vi "HFRR ADV v028 new software.vi"() -> ()   [LabVIEW 2025] (continued)
                      }
                      frame #27 {
                        n2418 = local read "Set Temp"() -> (w3472:dbl)
                        n2419 = Number To Fractional String(number=w3472, precision (6)=i16 2) -> (F-format string=w3473:string)  [unwired: 2 in]
                        n2420 = Concatenate Strings("Set Temperature [deg C] :" ("Content"), w3473) -> (w3475:string)
                        n2421 = local read "EVENT LOG"() -> (w3477:string)
                        n2422 = call "Event Log.vi"("Content"=w3475, "EVENT LOG"=w3477) -> ("EVENT LOG"=w3476:string)  [unwired: 8 in, 1 out]
                        n2423 = local write "EVENT LOG"(w3476) -> ()
                      }
                      frame #28 {
                        n2424 = Wait (ms)(milliseconds to wait=u32 50) -> ()  [unwired: 1 out]
                      }
                      frame #29 {
                        n2425 = local read "Set Rh"() -> (w3480:dbl)
                        n2426 = Number To Fractional String(number=w3480, precision (6)=i16 2) -> (F-format string=w3481:string)  [unwired: 2 in]
                        n2427 = Concatenate Strings("Set Humidity [%RH] :" ("Content"), w3481) -> (w3483:string)
                        n2428 = local read "EVENT LOG"() -> (w3485:string)
                        n2429 = call "Event Log.vi"("Content"=w3483, "EVENT LOG"=w3485) -> ("EVENT LOG"=w3484:string)  [unwired: 8 in, 1 out]
                        n2430 = local write "EVENT LOG"(w3484) -> ()
                      }
                      frame #30 {
                        n2431 = Wait (ms)(milliseconds to wait=u32 50) -> ()  [unwired: 1 out]
                      }
                      frame #31 {
                        n2432 = local read "test time"() -> (w3488:dbl)
                        n2433 = Number To Fractional String(number=w3488, precision (6)=i16 1) -> (F-format string=w3489:string)  [unwired: 2 in]
                        n2434 = Concatenate Strings("Test Duration [mins] :" ("Content"), w3489) -> (w3491:string)
                        n2435 = local read "EVENT LOG"() -> (w3493:string)
                        n2436 = call "Event Log.vi"("Content"=w3491, "EVENT LOG"=w3493) -> ("EVENT LOG"=w3492:string)  [unwired: 8 in, 1 out]
                        n2437 = local write "EVENT LOG"(w3492) -> ()
                      }
                      frame #32 {
                        w3494 = dbl[] [] ("History Data")
                        w3495 = cluster{"y":dbl, dbl, "y":dbl}[] [] ("History Data")
                        w3496 = FALSE ("Visible")
                        n2438 = property on="Stroke ( mm )" class="WFChart (strict)"("History Data"=w3495) -> ()  [unwired: 2 in, 2 out]
                        n2439 = property on="Humidity ( %RH )" class="WFChart (strict)"("History Data"=w3494) -> ()  [unwired: 2 in, 2 out]
                        n2440 = property on="Temperature ( Deg C )" class="WFChart (strict)"("History Data"=w3494) -> ()  [unwired: 2 in, 2 out]
                        n2441 = property on="Electrical Contact Resistance ( % )" class="WFChart (strict)"("History Data"=w3494) -> ()  [unwired: 2 in, 2 out]
                        n2442 = property on="Coefficient of Friction" class="WFChart (strict)"("History Data"=w3494) -> ()  [unwired: 2 in, 2 out]
                        n2443 = property on="Frictional Force ( N )" class="WFChart (strict)"("History Data"=w3494) -> ()  [unwired: 2 in, 2 out]
                        n2444 = property on="Coefficient of Friction" class="WFChart (strict)"("History Data"=w3494) -> ()  [unwired: 2 in, 2 out]
                        n2445 = property on="Frictional Force ( N )" class="WFChart (strict)"("History Data"=w3494) -> ()  [unwired: 2 in, 2 out]
                        n2446 = property on="Electrical Contact Resistance ( % )" class="WFChart (strict)"("History Data"=w3494) -> ()  [unwired: 2 in, 2 out]
                        n2447 = property on="Humidity ( %RH )" class="WFChart (strict)"("History Data"=w3494) -> ()  [unwired: 2 in, 2 out]
                        n2448 = property on="Stroke ( mm )" class="WFChart (strict)"("History Data"=w3495) -> ()  [unwired: 2 in, 2 out]
                        n2449 = property on="Temperature ( Deg C )" class="WFChart (strict)"("History Data"=w3494) -> ()  [unwired: 2 in, 2 out]
                        n2450 = property on="Service Password Log" class="Str"("Visible"=w3496) -> ()  [unwired: 2 in, 2 out]
                        n2451 = property on="Password 3" class="Clust (strict)"("Visible"=w3496) -> ()  [unwired: 2 in, 2 out]
                      }
                    }
                    "TEST FILE NAM,E SAVED" <- TRUE ("TEST FILE NAM,E SAVED")
                  }
                }
              }
            }
          }
        }
        n2452 = local write "Test \nStatus"(w2886) -> ()
        n2453 = local write "Save"(w2886) -> ()
        n2454 = local read "Main Tab"() -> (w2880:T2)
        n2455 = case shown="True" w2883 {
          frame False {
            n2456 = local read "Rt 3"() -> (w2955:bool)
            n2457 = case shown="True" w2955 {
              frame False {
              }
              frame True {
                n2458 = local write "Rt 3"(FALSE ("Rt 3")) -> ()
              }
            }
            "Rt" <- TRUE ("Rt")
            "Rt 2" <- FALSE ("Rt")
          }
          frame True {
            n2459 = local read "Rt"() -> (w2961:bool)
            n2460 = local write "Rt 2"(TRUE ("Rt 2")) -> ()
            n2461 = case shown="True" w2961 {
              frame False {
              }
              frame True {
                n2462 = local write "Rt"(FALSE ("Rt")) -> ()
              }
            }
            "Rt 3" <- TRUE ("Rt 3")
          }
        }
        n2463 = case shown="\"Acquire\"" w2880 {
          tunnel: w2882 -> [_ w2989]
          frame Default {
            w2988 = 0.0 ("output")
            n2464 = local write "PID-out"(w2988) -> ()
            n2465 = local write "Frequency ( Hz )"(w2988) -> ()
          }
          frame "Acquire" {
            n2466 = stacked-sequence {
              frame #0 {
                n2467 = local read "Auto Start Test"() -> (w2991:bool)
                n2468 = case shown="True" w2991 {
                  tunnel: "RUN" -> [w3012 w3015]
                  tunnel: [w3012 w3014] -> w2992
                  frame False {
                  }
                  frame True {
                    n2469 = local read "Auto Start Temp"() -> (w3013:bool)
                    n2470 = Or(x=w3015, y=w3013) -> (x .or. y?=w3014:bool)
                  }
                }
                n2471 = local read "clk"() -> (w3011:dbl)
                n2472 = local read "Save"() -> (w3007:bool)
                n2473 = Equal?(x=w3011, y=0.0) -> (x = y?=w3008:bool)
                n2474 = And(x=w3008, y=w3007) -> (x .and. y?=w3009:bool)
                n2475 = Not(x="Engage") -> (.not. x?=w2998:bool)
                n2476 = case shown="False" w2992 {
                  tunnel: [0.0 w3038] -> w2994
                  frame False {
                    (unwired) TRUE ("Visible")
                    n2477 = local read "Auto Start Test"() -> (w3019:bool)
                    n2478 = local write "Start Time"(TRUE ("Start Time")) -> ()
                    n2479 = property on="Stroke 2" class="DigNum (strict)"("Visible"=FALSE) -> ()  [unwired: 2 in, 2 out]
                    n2480 = case shown="False" w3019 {
                      frame False {
                        n2481 = property on="Heater Button" class="Bool (strict)"("DisabledEnum"=T19."Enabled" ("Disabled")) -> ()  [unwired: 2 in, 2 out]
                        n2482 = property on="Humidity" class="Bool (strict)"("DisabledEnum"=T19."Enabled" ("Disabled")) -> ()  [unwired: 2 in, 2 out]
                      }
                      frame True {
                      }
                    }
                    n2483 = case shown="False" "TestCompFlg" {
                      frame False {
                        n2484 = local read "StartFlg"() -> (w3027:bool)
                        n2485 = case shown="True" w3027 {
                          frame False {
                          }
                          frame True {
                            n2486 = stacked-sequence {
                              frame #0 {
                                n2487 = local read "EVENT LOG"() -> (w3031:string)
                                n2488 = call "Event Log.vi"("Content"="Test was interrupted", "EVENT LOG"=w3031) -> ("EVENT LOG"=w3032:string)  [unwired: 8 in, 1 out]
                                n2489 = local write "EVENT LOG"(w3032) -> ()
                                n2490 = property on="RUN" class="Bool (strict)"("Visible"=TRUE) -> ()  [unwired: 2 in, 2 out]
                                n2491 = property on="Auto Start Test" class="Bool (strict)"("Visible"=TRUE) -> ()  [unwired: 2 in, 2 out]
                              }
                              frame #1 {
                                w3034 = FALSE ("StartFlg")
                                n2492 = property on="Heater Button" class="Bool (strict)"("Val(Sgnl)"=FALSE ("Value (Signaling)")) -> ()  [unwired: 2 in, 2 out]
                                n2493 = local write "Heater Button"(w3034) -> ()
                                n2494 = local write "StartFlg"(w3034) -> ()
                                n2495 = local write "Humidity"(w3034) -> ()
                              }
                              frame #2 {
                                n2496 = local write "Due Write"("VC;0" ("Command")) -> ()
                              }
                              frame #3 {
                                n2497 = Wait (ms)(milliseconds to wait=u32 1500) -> ()  [unwired: 1 out]
                              }
                              frame #4 {
                                n2498 = local write "Due Write"("HE;0" ("Command")) -> ()
                              }
                            }
                          }
                        }
                      }
                      frame True {
                      }
                    }
                    n2499 = local write "String 14"("Test will autostart once parameters reach the set value." ("String 14")) -> ()
                  }
                  frame True {
                    (unwired) FALSE ("Visible")
                    n2500 = property on="Stroke 2" class="DigNum (strict)"("Visible"=TRUE) -> ()  [unwired: 2 in, 2 out]
                    n2501 = property on="STOP 2" class="Bool (strict)"("Disabled"=u8 2) -> ()  [unwired: 2 in, 2 out]
                    n2502 = local write "String 14"(" Running....." ("String 14")) -> ()
                    n2503 = property on="Heater Button" class="Bool (strict)"("DisabledEnum"=T19."Disabled and Grayed Out" ("Disabled")) -> ()  [unwired: 2 in, 2 out]
                    n2504 = property on="Humidity" class="Bool (strict)"("DisabledEnum"=T19."Disabled and Grayed Out" ("Disabled")) -> ()  [unwired: 2 in, 2 out]
                    n2505 = case shown="True" "Start Time" {
                      selector: "Start Time" -> [_ w3057]
                      frame False {
                      }
                      frame True {
                        n2506 = Not(x=w3057) -> (.not. x?=w3056:bool)
                        n2507 = local write "Start Time"(w3056) -> ()
                        n2508 = local read "EVENT LOG"() -> (w3058:string)
                        n2509 = call "Event Log.vi"("Content"="Test in progress", "EVENT LOG"=w3058) -> ("EVENT LOG"=w3060:string)  [unwired: 8 in, 1 out]
                        n2510 = local write "EVENT LOG"(w3060) -> ()
                      }
                    }
                    n2511 = disable-structure shown="Enabled" {
                      disable-tunnel: [w3049 w3055] -> w3038
                      frame Disabled {
                        n2512 = local read "Set Hz"() -> (w3052:dbl)
                        n2513 = call <vilib>:"Uniform White Noise Waveform.vi"() -> ("signal out"=w3051:waveform(dbl))  [unwired: 10 in, 1 out]
                        n2514 = Random Number (0-1)() -> (number: 0 to 1=w3048:dbl)
                        n2515 = Add(x=w3052, y=w3051) -> (x+y=w3050:waveform(dbl))
                        n2516 = Multiply(x=ext 0.01 ("y"), y=w3048) -> (x*y=w3046:ext)
                        n2517 = Multiply(x=w3050, y=w3046) -> (x*y=w3049:waveform(ext))
                      }
                      frame Enabled {
                        n2518 = call-poly <vilib>:"Random Number (Range).vi"("lower bound (0)"=49.89, "upper bound (100)"=50.8) -> ("number"=w3055:dbl)  [unwired: 9 in]
                      }
                    }
                    "StartFlg" <- TRUE ("StartFlg")
                  }
                }
                n2519 = case shown="True" w3009 {
                  frame False {
                  }
                  frame True {
                    n2520 = local write "clk"(10.0 ("clk")) -> ()
                    n2521 = Get Date/Time In Seconds() -> (seconds since 1Jan1904=w3063:timestamp)
                    n2522 = To Double Precision Float(number=w3063) -> (double precision float=w3061:dbl)
                    n2523 = local write "acq timer"(w3061) -> ()
                    n2524 = local write "act save time"(w3061) -> ()
                  }
                }
                n2525 = call "Elapsed Time"("Time Target (s)"="Countdown", "Reset"=w2998) -> ("Elapsed Time (s)"=w3003:dbl, "Time has Elapsed"=w3001:bool)  [unwired: 10 in, 6 out]
                "Countdown 2" <- w3003
                n2526 = Subtract(x=w3003, y=2.0) -> (x-y=w3006:dbl)
                n2527 = Less?(x=w3006, y="Countdown") -> (x < y?=w3004:bool)
                n2528 = And(x=w3004, y=w3001) -> (x .and. y?=w3000:bool)
                n2529 = case shown="True" w3000 {
                  frame False {
                  }
                  frame True {
                    (unwired) dbl[] [] ("History Data")
                    n2530 = local write "Engage"(FALSE ("Engage")) -> ()
                    n2531 = local write "RUN"(TRUE ("RUN")) -> ()
                    n2532 = local read "Humidity ( %RH )"() -> (→"Rh Before":dbl)
                  }
                }
                n2533 = local read "Test \nStatus"() -> (w2996:bool)
                n2534 = Select(t=w2994, s=w2996, f=0.0) -> (s? t:f=w2995:dbl)
                n2535 = local write "Frequency ( Hz )"(w2995) -> ()
              }
              frame #1 {
                w3086 = 1000000.0 ("x")
                # "HC;1/0\nST;VALUE"
                # "Elapsed time\ncof\nstroke\nAir temp\nTemp\nHumidity"
                # "acq timer\n\nact save time"
                # "convert to microseconds"
                n2536 = local read "COUNT"() -> (w3069:i32)
                n2537 = local read "Rate"() -> (w3082:dbl)
                n2538 = Divide(x=w3086, y=w3082) -> (x/y=w3087:dbl)
                n2539 = Greater Or Equal?(x=w3069, y=250) -> (x >= y?=w3068:bool)
                n2540 = Get Date/Time In Seconds() -> (seconds since 1Jan1904=w3089:timestamp)
                n2541 = case shown="True" w3068 {
                  frame False {
                    n2542 = local read "COUNT"() -> (w3090:i32)
                    n2543 = Increment(x=w3090) -> (x+1=w3091:i32)
                    n2544 = local write "COUNT"(w3091) -> ()
                  }
                  frame True {
                    n2545 = local write "COUNT"(0 ("COUNT")) -> ()
                  }
                }
                n2546 = local read "Samplingtime 2"() -> (w3067:dbl)
                n2547 = local read "act save time"() -> (w3084:dbl)
                n2548 = Divide(x=w3087, y=w3086) -> (x/y=w3085:dbl)
                n2549 = To Double Precision Float(number=w3089) -> (double precision float=w3078:dbl)
                n2550 = Add(x=w3084, y=w3067) -> (x+y=w3083:dbl)
                n2551 = local read "acq timer"() -> (w3088:dbl)
                n2552 = local read "COUNT"() -> (w3071:i32)
                n2553 = Greater Or Equal?(x=w3078, y=w3083) -> (x >= y?=w3066:bool)
                n2554 = Multiply(x=w3085, y=w3071) -> (x*y=w3077:dbl)
                n2555 = Subtract(x=w3078, y=w3088) -> (x-y=w3080:dbl)
                n2556 = local read "Save"() -> (w3081:bool)
                n2557 = Add(x=w3080, y=w3077) -> (x+y=w3064:dbl)
                "Elapsed time 3" <- w3064
                n2558 = And(x=w3066, y=w3081) -> (x .and. y?=w3079:bool)
                n2559 = Divide(x=w3064, y=60.0) -> (x/y=w3075:dbl)
                n2560 = local read "Test \nStatus"() -> (w3065:bool)
                n2561 = local read "clk"() -> (w3072:dbl)
                n2562 = Equal?(x=w3072, y=10.0) -> (x = y?=w3074:bool)
                n2563 = case shown="True" w3079 {
                  tunnel: w3078 -> [_ w3202]
                  tunnel: [FALSE ("Boolean 2") TRUE ("Boolean 2")] -> _
                  frame False {
                  }
                  frame True {
                    w3156 = ";" ("Substring")
                    # "Pid out/\nFreq response value"
                    n2564 = local write "act save time"(w3202) -> ()
                    n2565 = local read "FILE"() -> (w3150:string)
                    n2566 = call "file check.vi"("file name in"=w3150) -> ("error out"=w3153:errorcluster, "file name out"=w3148:string)  [unwired: 9 in]
                    n2567 = local read "LVDT STROKE"() -> (w3145:dbl)
                    n2568 = local read "Add up Stroke"() -> (w3143:dbl)
                    n2569 = call "FILE PATH CREATION.vi"("error in"=w3153, "FILE NAME :"=w3148) -> ("FILE OUT"=w3151:path)  [unwired: 8 in, 1 out]
                    n2570 = Concatenate Strings(w3148, ".dgf" ("Substring")) -> (w3152:string)
                    n2571 = Subtract(x=w3145, y=w3143) -> (x-y=w3144:dbl)
                    n2572 = Absolute Value(x=w3144) -> (abs(x)=w3142:dbl)
                    n2573 = local read "FF 2"() -> (→"Frictional Force ( N )" →"Frictional Force ( N )":dbl)
                    n2574 = Build Path(base path=w3151, name or relative path=w3152) -> (appended path=w3147:path)
                    n2575 = local read "COF 2"() -> (w3161:dbl)
                    "Coefficient of Friction" <- w3161
                    "COF 4" <- w3161
                    "Coefficient of Friction" <- w3161
                    n2576 = local read "TEMP"() -> (w3164:dbl)
                    "Temperature ( Deg C )" <- w3164
                    n2577 = local read "Humidity ( %RH )"() -> (w3163:dbl)
                    "Humidity ( %RH )" <- w3163
                    "Humidity ( %RH )" <- w3163
                    n2578 = local read "Frequency ( Hz )"() -> (w3170:dbl)
                    n2579 = call <vilib>:"Mean PtByPt.vi"("x"=w3142, "sample length"="STROKE FILTER") -> ("mean"=w3141:dbl)  [unwired: 2 in, 1 out]
                    n2580 = local read "Elapsed time"() -> (w3195:dbl)
                    n2581 = local read "AIR TEMP"() -> (w3168:dbl)
                    n2582 = local read "PID-out"() -> (w3173:dbl)
                    n2583 = local write "Temperature ( Deg C )"(w3164) -> ()
                    n2584 = Number To Fractional String(number=w3141, width (-)=i16 9 ("precision (6)"), precision (6)=i16 6) -> (F-format string=w3188:string)  [unwired: 1 in]
                    n2585 = Number To Fractional String(number=w3168, width (-)=i16 9 ("precision (6)"), precision (6)=i16 3) -> (F-format string=w3187:string)  [unwired: 1 in]
                    n2586 = Number To Fractional String(number=w3164, width (-)=i16 9 ("precision (6)"), precision (6)=i16 3) -> (F-format string=w3184:string)  [unwired: 1 in]
                    n2587 = Number To Fractional String(number=w3163, width (-)=i16 9 ("precision (6)"), precision (6)=i16 3) -> (F-format string=w3181:string)  [unwired: 1 in]
                    n2588 = Number To Fractional String(number=0.0, width (-)=i16 9 ("precision (6)"), precision (6)=i16 3) -> (F-format string=w3178:string)  [unwired: 1 in]
                    n2589 = Number To Fractional String(number=w3173, width (-)=i16 9 ("precision (6)"), precision (6)=i16 3) -> (F-format string=w3174:string)  [unwired: 1 in]
                    n2590 = Number To Fractional String(number=w3170, width (-)=i16 9 ("precision (6)"), precision (6)=i16 3) -> (F-format string=w3169:string)  [unwired: 1 in]
                    n2591 = Number To Fractional String(number=w3161, width (-)=i16 9 ("precision (6)"), precision (6)=i16 6) -> (F-format string=w3196:string)  [unwired: 1 in]
                    n2592 = Number To Fractional String(number=w3195, width (-)=i16 14 ("precision (6)"), precision (6)=i16 3) -> (F-format string=w3197:string)  [unwired: 1 in]
                    n2593 = Bundle("y"=1.02, "mean"=w3141, "y"=0.98) -> (w3162:cluster{"y":dbl, "mean":dbl, "y":dbl})  [unwired: 1 in]
                    n2594 = Number To Fractional String(number="Ambient Humidity :", width (-)=i16 9 ("precision (6)"), precision (6)=i16 6) -> (F-format string=w3154:string)  [unwired: 1 in]
                    n2595 = local read "RUN"() -> (w3160:bool)
                    n2596 = case shown="True" w3160 {
                      tunnel: w3162 -> [_ w3207]
                      tunnel: w3141 -> [_ w3206]
                      tunnel: w3141 -> [_ w3204]
                      tunnel: w3141 -> [_ w3205]
                      frame False {
                      }
                      frame True {
                        "Stroke ( mm )" <- w3207
                        "Stroke ( mm )" <- w3207
                        "Stroke 4" <- w3206
                        "Stroke 3" <- w3204
                        "Stroke 2" <- w3205
                        "measured_stroke" <- w3204
                      }
                    }
                    n2597 = Concatenate Strings(w3197, w3156, w3196, w3156, w3188, w3156, w3187, w3156, w3184, w3156, w3181, w3156, w3178, w3156, w3174, w3156, w3169, w3156, w3154, "\r") -> (w3194:string)
                    n2598 = call <vilib>:"Write Characters To File.vi"("append to file? (new file:F)"=TRUE, "character string"=w3194, "file path (dialog if empty)"=w3147) -> ()  [unwired: 2 in, 1 out]
                    "refresh flag" <- TRUE ("refresh flag")
                  }
                }
                n2599 = case shown="True" w3065 {
                  tunnel: w3075 -> [_ w3101]
                  tunnel: w3080 -> [_ w3111]
                  tunnel: [0.0 w3107] -> _
                  tunnel: w3074 -> [_ w3106]
                  tunnel: [0.0 w3105] -> _
                  tunnel: w3064 -> [_ w3105]
                  tunnel: w3078 -> [w3094 _]
                  frame False {
                    n2600 = local write "acq timer"(w3094) -> ()
                    n2601 = local write "Test Duration Status"(0.0 ("Test Duration Status")) -> ()
                  }
                  frame True {
                    n2602 = local read "Set Hz"() -> (w3108:dbl)
                    n2603 = local write "Elapsed time"(w3101) -> ()
                    n2604 = local read "test time"() -> (w3100:dbl)
                    n2605 = Multiply(x=w3111, y=w3108) -> (x*y=w3110:dbl)
                    n2606 = case shown="False" w3106 {
                      tunnel: w3110 -> [w3112 _]
                      tunnel: [w3112 1.0] -> w3107
                      frame False {
                        n2607 = local write "Cycles elapsed"(w3112) -> ()
                      }
                      frame True {
                      }
                    }
                    n2608 = Greater?(x=w3101, y=w3100) -> (0:w3109:bool)
                    n2609 = Subtract(x=w3100, y=w3101) -> (x-y=w3099:dbl)
                    n2610 = Multiply(x=w3099, y=60.0) -> (x*y=w3098:dbl)
                    n2611 = local write "Time Remaining"(w3098) -> ()
                    n2612 = local write "Remaining Time"(w3098) -> ()
                    n2613 = case shown="True" w3109 {
                      frame False {
                      }
                      frame True {
                        n2614 = stacked-sequence {
                          frame #0 {
                            w3117 = T19."Enabled" ("Disabled")
                            w3116 = FALSE ("TEST FILE NAM,E SAVED")
                            w3118 = "" ("FILE")
                            w3119 = TRUE ("Visible")
                            n2615 = local write "Humidity"(FALSE ("Humidity")) -> ()
                            n2616 = local write "RUN"(FALSE ("OK Button 2")) -> ()
                            n2617 = local write "Heater Button"(FALSE ("Heater Button")) -> ()
                            n2618 = local write "Auto Start Test"(FALSE ("Auto Start Test")) -> ()
                            n2619 = local write "TestCompFlg"(TRUE ("StpFlg")) -> ()
                            n2620 = local read "Humidity ( %RH )"() -> (→"Rh After":dbl)
                            n2621 = property on="STOP 2" class="Bool (strict)"("Disabled"=u8 0) -> ()  [unwired: 2 in, 2 out]
                            n2622 = local read "EVENT LOG"() -> (w3124:string)
                            n2623 = call "Event Log.vi"("Content"="Test Completed", "EVENT LOG"=w3124) -> ("EVENT LOG"=w3123:string)  [unwired: 8 in, 1 out]
                            n2624 = property on="RUN" class="Bool (strict)"("Visible"=w3119) -> ()  [unwired: 2 in, 2 out]
                            n2625 = property on="Auto Start Test" class="Bool (strict)"("Visible"=w3119) -> ()  [unwired: 2 in, 2 out]
                            n2626 = local write "Batch Ref Num :"(w3118) -> ()
                            n2627 = local write "FILE"(w3118) -> ()
                            n2628 = local write "EVENT LOG"(w3123) -> ()
                            n2629 = local write "TEST FILE NAM,E SAVED"(w3116) -> ()
                            n2630 = local write "Fuel Discription :"(w3118) -> ()
                            n2631 = local write "START TEMP"(w3116) -> ()
                            n2632 = local write "Remarks :"(w3118) -> ()
                            n2633 = local write "Main Dashboard Buttons"(T1."Imaging" ("Main Dashboard Buttons")) -> ()
                            n2634 = local write "Main Tab"(T2."Adv Scar" ("Main Tab")) -> ()
                            n2635 = property on="FRICVALZ 2" class="Bool (strict)"("DisabledEnum"=w3117) -> ()  [unwired: 2 in, 2 out]
                            n2636 = property on="FRICVALZ 3" class="Bool (strict)"("DisabledEnum"=w3117) -> ()  [unwired: 2 in, 2 out]
                            n2637 = property on="FRICVALZ 4" class="Bool (strict)"("DisabledEnum"=w3117) -> ()  [unwired: 2 in, 2 out]
                          }
                          frame #1 {
                            n2638 = Wait (ms)(milliseconds to wait=u32 1500) -> ()  [unwired: 1 out]
                          }
                          frame #2 {
                            n2639 = local write "Due Write"("VC;0") -> ()
                          }
                          frame #3 {
                            n2640 = Wait (ms)(milliseconds to wait=u32 1500) -> ()  [unwired: 1 out]
                          }
                          frame #4 {
                            n2641 = local write "Due Write"("VC;0") -> ()
                          }
                          frame #5 {
                            n2642 = Wait (ms)(milliseconds to wait=u32 1500) -> ()  [unwired: 1 out]
                          }
                          frame #6 {
                            n2643 = local write "Due Write"("ST;0") -> ()
                          }
                          frame #7 {
                            n2644 = local write "measured_stroke"(0.0 ("measured_stroke")) -> ()
                            n2645 = Wait (ms)(milliseconds to wait=u32 1500) -> ()  [unwired: 1 out]
                          }
                          frame #8 {
                            n2646 = local write "Due Write"("HE;0") -> ()
                          }
                        }
                      }
                    }
                    n2647 = Divide(x=w3101, y=w3100) -> (x/y=w3104:dbl)
                    n2648 = Multiply(x=w3104, y=100.0) -> (x*y=w3102:dbl)
                    n2649 = local write "Test Duration Status"(w3102) -> ()
                  }
                }
              }
              frame #2 {
                n2650 = case shown="True" "Heater Button" {
                  tunnel: [0.0 ("output") w3230] -> w3208
                  frame False {
                    w3211 = TRUE ("tmpchk")
                    n2651 = local read "TEMP"() -> (w3212:dbl)
                    n2652 = local write "Temp ini"(w3212) -> ()
                    n2653 = local write "Reset 4"(w3211) -> ()
                    n2654 = local write "tmpchk"(w3211) -> ()
                    n2655 = local write "reinit"(TRUE ("reinit")) -> ()
                    n2656 = local write "manual temp log"(TRUE ("manual temp log")) -> ()
                  }
                  frame True {
                    # "Logic to turn off\nthe heater when \ntemp is not rising.\nTime - 60 sec\nDelta t- 5°c"
                    n2657 = local read "Temp ini"() -> (w3219:dbl)
                    n2658 = local read "Auto Start Test"() -> (w3215:bool)
                    n2659 = Less?(x=w3219, y=53.0) -> (x < y?=w3217:bool)
                    n2660 = case shown="False" w3215 {
                      frame False {
                        n2661 = local read "Set Temp"() -> (w3239:dbl)
                        n2662 = local read "TEMP"() -> (w3238:dbl)
                        n2663 = Subtract(x=w3239, y=w3238) -> (x-y=w3237:dbl)
                        n2664 = Absolute Value(x=w3237) -> (abs(x)=w3236:dbl)
                        n2665 = Less?(x=w3236, y=0.5) -> (x < y?=w3234:bool)
                        n2666 = case shown="True" w3234 {
                          tunnel: "manual temp log" -> [_ w3240]
                          frame False {
                          }
                          frame True {
                            n2667 = case shown="True" w3240 {
                              selector: w3240 -> [_ w3241]
                              frame False {
                              }
                              frame True {
                                # "#Event log"
                                n2668 = Not(x=w3241) -> (.not. x?=w3242:bool)
                                n2669 = local write "manual temp log"(w3242) -> ()
                                n2670 = local read "EVENT LOG"() -> (w3245:string)
                                n2671 = call "Event Log.vi"("Content"="Target Temperature reached", "EVENT LOG"=w3245) -> ("EVENT LOG"=w3244:string)  [unwired: 8 in, 1 out]
                                n2672 = local write "EVENT LOG"(w3244) -> ()
                              }
                            }
                          }
                        }
                      }
                      frame True {
                        n2673 = local write "manual temp log"(TRUE ("manual temp log")) -> ()
                      }
                    }
                    n2674 = And(x="tmpchk", y=w3217) -> (x .and. y?=w3220:bool)
                    n2675 = case shown="True" w3220 {
                      frame False {
                      }
                      frame True {
                        n2676 = call "Elapsed Time8"("Time Target (s)"=300.0, "Reset"="Reset 4") -> ("Time has Elapsed"=w3247:bool)  [unwired: 10 in, 7 out]
                        n2677 = flat-sequence {
                          tunnel: w3247 -> [_]
                          frame #0 {
                            n2678 = local write "Reset 4"(FALSE ("Reset 4")) -> ()
                          }
                        }
                        n2679 = case shown="True" w3247 {
                          frame False {
                          }
                          frame True {
                            n2680 = local read "Temp ini"() -> (w3254:dbl)
                            n2681 = Add(x=w3254, y=5.0) -> (x+y=w3252:dbl)
                            n2682 = local read "TEMP"() -> (w3255:dbl)
                            n2683 = Greater?(x=w3255, y=w3252) -> (0:w3253:bool)
                            n2684 = case shown="False" w3253 {
                              frame False {
                                n2685 = local write "Heater Button"(FALSE ("Heater Button")) -> ()
                              }
                              frame True {
                                n2686 = local write "tmpchk"(FALSE ("tmpchk")) -> ()
                              }
                            }
                          }
                        }
                      }
                    }
                    n2687 = local read "Set Temp"() -> (w3228:dbl)
                    n2688 = local read "TEMP"() -> (w3222:dbl)
                    n2689 = call-poly <vilib>:"PID.vi"("reinitialize? (F)"="reinit", "dt (s)"=-1.0, "process variable"=w3222, "setpoint"=w3228) -> ("output"=w3225:dbl)  [unwired: 6 in, 1 out]
                    n2690 = Subtract(x=w3228, y=w3222) -> (x-y=w3229:dbl)
                    n2691 = Add(x=w3228, y=0.5) -> (x+y=w3226:dbl)
                    n2692 = Greater Or Equal?(x=w3222, y=w3226) -> ()  [unwired: 1 out]
                    n2693 = Select(t=0.0, s=FALSE, f=w3225) -> (s? t:f=w3224:dbl)
                    "PID output" <- w3224
                    n2694 = flat-sequence {
                      tunnel: w3224 -> [w3258]
                      tunnel: [w3258] -> w3230
                      frame #0 {
                        n2695 = local write "reinit"(FALSE ("reinit")) -> ()
                      }
                    }
                    n2696 = Bundle(w3229, "output"=w3224, "TEMP"=w3222) -> ()  [unwired: 1 in, 1 out]
                  }
                }
                "PID-out" <- w3208
              }
              frame #3 {
                n2697 = local read "TEMP"() -> (w3260:dbl)
                n2698 = Greater Or Equal?(x=w3260, y="Set Temp 2") -> (x >= y?=w3265:bool)
                n2699 = case shown="True" w3265 {
                  tunnel: [FALSE TRUE] -> w3263
                  frame False {
                  }
                  frame True {
                  }
                }
                "Status 13" <- w3263
                n2700 = And(x=w3263, y="trip1 8") -> (x .and. y?=w3262:bool)
                n2701 = case shown="True" w3262 {
                  frame False {
                    n2702 = local write "Heater Trip Temp"(TRUE ("Heater Trip Temp")) -> ()
                  }
                  frame True {
                    w3268 = FALSE ("OK Button 2")
                    n2703 = case shown="True" "Heater Trip Temp" {
                      selector: "Heater Trip Temp" -> [_ w3270]
                      frame False {
                      }
                      frame True {
                        n2704 = Not(x=w3270) -> (.not. x?=w3269:bool)
                        n2705 = local read "EVENT LOG"() -> (w3273:string)
                        n2706 = local write "Heater Trip Temp"(w3269) -> ()
                        n2707 = call "Event Log.vi"("Content"="Heater Trip", "EVENT LOG"=w3273) -> ("EVENT LOG"=w3272:string)  [unwired: 8 in, 1 out]
                        n2708 = local write "EVENT LOG"(w3272) -> ()
                      }
                    }
                    n2709 = local write "RUN"(w3268) -> ()
                    n2710 = property on="Auto Start Test" class="Bool (strict)"("Value"=w3268) -> ()  [unwired: 2 in, 2 out]
                    n2711 = local write "Heater Button"(w3268) -> ()
                  }
                }
              }
            }
            n2712 = case shown="False" w2989 {
              frame False {
                n2713 = disable-structure shown="Disabled" {
                  frame Disabled {
                    n2714 = stacked-sequence {
                      frame #0 {
                        n2715 = local write "RUN"(FALSE ("OK Button 2")) -> ()
                      }
                      frame #1 {
                      }
                    }
                  }
                  frame Enabled {
                  }
                }
              }
              frame True {
              }
            }
          }
        }
        n2716 = local read "Reset Graph"() -> (w2879:bool)
        n2717 = case shown="True" w2879 {
          selector: w2879 -> [_ w2896]
          frame False {
          }
          frame True {
            w2910 = 0.0 ("X Scale.Range:Maximum")
            n2718 = Not(x=w2896) -> (.not. x?=w2895:bool)
            n2719 = local write "Reset Graph"(w2895) -> ()
            n2720 = property on="Electrical Contact Resistance ( % )" class="WFChart (strict)"("XScale.Maximum"=600.0 ("X Scale.Range:Maximum"), "XScale.Minimum"=0.0 ("X Scale.Range:Minimum"), "YScale.Maximum"=100.0 ("Y Scale.Range:Maximum"), "YScale.Minimum"=0.0 ("Y Scale.Range:Minimum")) -> ()  [unwired: 2 in, 2 out]
            n2721 = property on="Frictional Force ( N )" class="WFChart (strict)"("XScale.Maximum"=600.0 ("X Scale.Range:Maximum"), "XScale.Minimum"=0.0 ("X Scale.Range:Minimum"), "YScale.Maximum"=100.0 ("Y Scale.Range:Maximum"), "YScale.Minimum"=0.0 ("Y Scale.Range:Minimum")) -> ()  [unwired: 2 in, 2 out]
            n2722 = property on="Temperature ( Deg C )" class="WFChart (strict)"("XScale.Maximum"=600.0 ("X Scale.Range:Maximum"), "XScale.Minimum"=0.0 ("X Scale.Range:Minimum"), "YScale.Maximum"=100.0 ("Y Scale.Range:Maximum"), "YScale.Minimum"=0.0 ("Y Scale.Range:Minimum")) -> ()  [unwired: 2 in, 2 out]
            n2723 = property on="Humidity ( %RH )" class="WFChart (strict)"("XScale.Maximum"=600.0 ("X Scale.Range:Maximum"), "XScale.Minimum"=0.0 ("X Scale.Range:Minimum"), "YScale.Maximum"=100.0 ("Y Scale.Range:Maximum"), "YScale.Minimum"=0.0 ("Y Scale.Range:Minimum")) -> ()  [unwired: 2 in, 2 out]
            n2724 = property on="Stroke ( mm )" class="WFChart (strict)"("XScale.Maximum"=600.0 ("X Scale.Range:Maximum"), "XScale.Minimum"=0.0 ("X Scale.Range:Minimum"), "YScale.Maximum"=100.0 ("Y Scale.Range:Maximum"), "YScale.Minimum"=0.0 ("Y Scale.Range:Minimum")) -> ()  [unwired: 2 in, 2 out]
            n2725 = property on="Coefficient of Friction" class="WFChart (strict)"("XScale.Maximum"=600.0 ("X Scale.Range:Maximum"), "XScale.Minimum"=0.0 ("X Scale.Range:Minimum"), "YScale.Maximum"=100.0 ("Y Scale.Range:Maximum"), "YScale.Minimum"=0.0 ("Y Scale.Range:Minimum")) -> ()  [unwired: 2 in, 2 out]
            n2726 = property on="Electrical Contact Resistance ( % )" class="WFChart (strict)"("XScale.Minimum"=0.0 ("X Scale.Range:Minimum"), "XScale.Maximum"=600.0 ("X Scale.Range:Maximum"), "YScale.Minimum"=0.0 ("Y Scale.Range:Minimum"), "YScale.Maximum"=100.0 ("Y Scale.Range:Maximum")) -> ()  [unwired: 2 in, 2 out]
            n2727 = property on="Temperature ( Deg C )" class="WFChart (strict)"("XScale.Minimum"=0.0 ("X Scale.Range:Minimum"), "XScale.Maximum"=600.0 ("X Scale.Range:Maximum"), "YScale.Minimum"=0.0 ("Y Scale.Range:Minimum"), "YScale.Maximum"=100.0 ("Y Scale.Range:Maximum")) -> ()  [unwired: 2 in, 2 out]
            n2728 = property on="Coefficient of Friction" class="WFChart (strict)"("XScale.Minimum"=0.0 ("X Scale.Range:Minimum"), "XScale.Maximum"=600.0 ("X Scale.Range:Maximum"), "YScale.Maximum"=1.0 ("X Scale.Range:Minimum"), "YScale.Minimum"=0.0 ("X Scale.Range:Minimum")) -> ()  [unwired: 2 in, 2 out]
            n2729 = property on="Frictional Force ( N )" class="WFChart (strict)"("XScale.Maximum"=600.0 ("X Scale.Range:Maximum"), "XScale.Minimum"=w2910, "YScale.Maximum"=10.0 ("Y Scale.Range:Maximum"), "YScale.Minimum"=w2910) -> ()  [unwired: 2 in, 2 out]
            n2730 = property on="Stroke ( mm )" class="WFChart (strict)"("XScale.Maximum"=600.0 ("X Scale.Range:Maximum"), "XScale.Minimum"=0.0 ("X Scale.Range:Minimum"), "YScale.Maximum"=100.0 ("Y Scale.Range:Maximum"), "YScale.Minimum"=0.0 ("Y Scale.Range:Minimum")) -> ()  [unwired: 2 in, 2 out]
            n2731 = property on="Humidity ( %RH )" class="WFChart (strict)"("XScale.Maximum"=600.0 ("X Scale.Range:Maximum"), "XScale.Minimum"=0.0 ("X Scale.Range:Minimum"), "YScale.Maximum"=100.0 ("Y Scale.Range:Maximum"), "YScale.Minimum"=0.0 ("Y Scale.Range:Minimum")) -> ()  [unwired: 2 in, 2 out]
          }
        }
      }
      frame "Compare Files" {
        # "Elapsed time\ncof\nstroke\nAir temp\nTemp\nHumidity"
        n2732 = case shown="True" "RSTV1 2" {
          frame False {
          }
          frame True {
            n2733 = property on="Humidity ( %RH )" class="XYGraph (strict)"("Y Scale.Display Format:Precision"=u8 0 ("Y Scale.Format & Precision:Precision")) -> ()  [unwired: 2 in, 2 out]
            n2734 = property on="Humidity ( %RH )" class="XYGraph (strict)"("X Scale.Range:Minimum"=0.0, "X Scale.Range:Maximum"=75.0, "Y Scale.Range:Minimum"=48.0, "Y Scale.Range:Maximum"=58.0) -> ()  [unwired: 2 in, 2 out]
          }
        }
        n2735 = case shown="True" "RST CP 2" {
          frame False {
          }
          frame True {
            n2736 = property on="XY Graph 13" class="XYGraph (strict)"("Y Scale.Display Format:Precision"=u8 0 ("Y Scale.Format & Precision:Precision")) -> ()  [unwired: 2 in, 2 out]
            n2737 = property on="XY Graph 13" class="XYGraph (strict)"("X Scale.Range:Minimum"=0.0, "X Scale.Range:Maximum"=75.0, "Y Scale.Range:Minimum"=0.0, "Y Scale.Range:Maximum"=100.0) -> ()  [unwired: 2 in, 2 out]
          }
        }
        n2738 = case shown="True" "RST CP" {
          frame False {
          }
          frame True {
            n2739 = property on="Sample Temperature ( °C )" class="XYGraph (strict)"("Y Scale.Display Format:Precision"=u8 2 ("Y Scale.Format & Precision:Precision")) -> ()  [unwired: 2 in, 2 out]
            n2740 = property on="Sample Temperature ( °C )" class="XYGraph (strict)"("X Scale.Range:Minimum"=0.0, "X Scale.Range:Maximum"=75.0, "Y Scale.Range:Minimum"=58.0, "Y Scale.Range:Maximum"=62.0) -> ()  [unwired: 2 in, 2 out]
          }
        }
        n2741 = case shown="True" "RSTV1 3" {
          frame False {
          }
          frame True {
            n2742 = property on="Air Temperature  ( °C )" class="XYGraph (strict)"("Y Scale.Display Format:Precision"=u8 2 ("Y Scale.Format & Precision:Precision")) -> ()  [unwired: 2 in, 2 out]
            n2743 = property on="Air Temperature  ( °C )" class="XYGraph (strict)"("X Scale.Range:Minimum"=0.0 ("Y Scale.Range:Minimum"), "X Scale.Range:Maximum"=75.0 ("Y Scale.Range:Maximum"), "Y Scale.Range:Minimum"=20.0 ("X Scale.Range:Minimum"), "Y Scale.Range:Maximum"=26.0 ("X Scale.Range:Maximum")) -> ()  [unwired: 2 in, 2 out]
          }
        }
        n2744 = case shown="True" "RSTV1 4" {
          frame False {
          }
          frame True {
            n2745 = property on="Stroke ( mm )" class="XYGraph (strict)"("Y Scale.Display Format:Precision"=u8 2 ("Y Scale.Format & Precision:Precision")) -> ()  [unwired: 2 in, 2 out]
            n2746 = property on="Stroke ( mm )" class="XYGraph (strict)"("X Scale.Range:Minimum"=0.0 ("Y Scale.Range:Maximum"), "X Scale.Range:Maximum"=75.0 ("X Scale.Range:Minimum"), "Y Scale.Range:Minimum"=0.98, "Y Scale.Range:Maximum"=1.02) -> ()  [unwired: 2 in, 2 out]
          }
        }
        n2747 = case shown="True" "rstv2" {
          frame False {
          }
          frame True {
            n2748 = property on="Coefficient Of Friction" class="XYGraph (strict)"("Y Scale.Display Format:Precision"=u8 3 ("Y Scale.Format & Precision:Precision")) -> ()  [unwired: 2 in, 2 out]
            n2749 = property on="Coefficient Of Friction" class="XYGraph (strict)"("X Scale.Range:Minimum"=0.0 ("Y Scale.Range:Maximum"), "X Scale.Range:Maximum"=75.0, "Y Scale.Range:Minimum"=0.0, "Y Scale.Range:Maximum"=1.0 ("X Scale.Range:Minimum")) -> ()  [unwired: 2 in, 2 out]
          }
        }
        n2750 = case shown="True" "RST CP 3" {
          frame False {
          }
          frame True {
            n2751 = property on="Air Temp ( °C ) vs Humidity ( % RH )" class="XYGraph (strict)"("X Scale.Range:Minimum"=18.0, "X Scale.Range:Maximum"=28.0 ("X Scale.Range:Minimum"), "Y Scale.Range:Minimum"=30.0 ("X Scale.Range:Minimum"), "Y Scale.Range:Maximum"=70.0 ("X Scale.Range:Minimum")) -> ()  [unwired: 2 in, 2 out]
          }
        }
        n2752 = case shown="True" "OPEN 1" {
          frame False {
          }
          frame True {
            (unwired) 0  # existing file
            w3549 = "Choose a datalog file to open"  # prompt
            n2753 = local write "OPEN 1"(FALSE ("OPEN 1")) -> ()
            n2754 = String To Path(string="C:\\LAB-IQ\\Data\\") -> (path=w3534:path)
            n2755 = File Dialog(6:"*.dgf" ("pattern"), 7:w3549, 11:w3534) -> (0:w3532:errorcluster, 3:w3540:path)  [unwired: 4 in, 2 out]
            n2756 = Unbundle(w3532) -> ()  [unwired: 3 out]
            n2757 = Strip Path(path=w3540) -> (name=w3539:string)  [unwired: 1 out]
            n2758 = Path To String(path=w3540) -> (string=w3535:string)
            "string1" <- w3535
            n2759 = Match Pattern(string=w3539, regular expression=".dgf") -> (before substring=→"String Control":string)  [unwired: 1 in, 3 out]
            n2760 = Match Pattern(string=w3535, regular expression=".dgf" ("substring (\"\")")) -> (before substring=w3545:string)  [unwired: 1 in, 3 out]
            n2761 = Concatenate Strings(w3545, ".duf" ("Substring")) -> (w3541:string)
            n2762 = String To Path(string=w3541) -> (path=w3546:path)
            n2763 = call <vilib>:"Read Characters From File.vi"("file path (dialog if empty)"=w3546, "start of read offset (chars.:0)"=60 ("start of read offset (chars.: 0)")) -> ("character string"=→"String Control 2":string)  [unwired: 4 in, 3 out]
          }
        }
        n2764 = case shown="True" "OPEN 2" {
          frame False {
          }
          frame True {
            (unwired) 0  # existing file
            w3567 = "Choose a datalog file to open"  # prompt
            n2765 = local write "OPEN 2"(FALSE ("OPEN 1")) -> ()
            n2766 = String To Path(string="C:\\LAB-IQ\\Data\\") -> (path=w3552:path)
            n2767 = File Dialog(6:"*.dgf" ("pattern"), 7:w3567, 11:w3552) -> (0:w3550:errorcluster, 3:w3558:path)  [unwired: 4 in, 2 out]
            n2768 = Unbundle(w3550) -> ()  [unwired: 3 out]
            n2769 = Strip Path(path=w3558) -> (name=w3556:string)  [unwired: 1 out]
            n2770 = Path To String(path=w3558) -> (string=w3553:string)
            "string1 2" <- w3553
            n2771 = Match Pattern(string=w3556, regular expression=".dgf") -> (before substring=→"String Control 3":string)  [unwired: 1 in, 3 out]
            n2772 = Match Pattern(string=w3553, regular expression=".dgf" ("substring (\"\")")) -> (before substring=w3564:string)  [unwired: 1 in, 3 out]
            n2773 = Concatenate Strings(w3564, ".duf" ("Substring")) -> (w3561:string)
            n2774 = String To Path(string=w3561) -> (path=w3559:path)
            n2775 = call <vilib>:"Read Characters From File.vi"("file path (dialog if empty)"=w3559, "start of read offset (chars.:0)"=60 ("start of read offset (chars.: 0)")) -> ("character string"=→"String Control 4":string)  [unwired: 4 in, 3 out]
          }
        }
        n2776 = case shown="True" "OPEN 3" {
          frame False {
          }
          frame True {
            (unwired) 0  # existing file
            w3585 = "Choose a datalog file to open"  # prompt
            n2777 = local write "OPEN 3"(FALSE ("OPEN 1")) -> ()
            n2778 = String To Path(string="C:\\LAB-IQ\\Data\\") -> (path=w3570:path)
            n2779 = File Dialog(6:"*.dgf" ("pattern"), 7:w3585, 11:w3570) -> (0:w3568:errorcluster, 3:w3576:path)  [unwired: 4 in, 2 out]
            n2780 = Unbundle(w3568) -> ()  [unwired: 3 out]
            n2781 = Strip Path(path=w3576) -> (name=w3574:string)  [unwired: 1 out]
            n2782 = Path To String(path=w3576) -> (string=w3571:string)
            "string1 3" <- w3571
            n2783 = Match Pattern(string=w3574, regular expression=".dgf") -> (before substring=→"String Control 5":string)  [unwired: 1 in, 3 out]
            n2784 = Match Pattern(string=w3571, regular expression=".dgf" ("substring (\"\")")) -> (before substring=w3581:string)  [unwired: 1 in, 3 out]
            n2785 = Concatenate Strings(w3581, ".duf" ("Substring")) -> (w3578:string)
            n2786 = String To Path(string=w3578) -> (path=w3582:path)
            n2787 = call <vilib>:"Read Characters From File.vi"("file path (dialog if empty)"=w3582, "start of read offset (chars.:0)"=60 ("start of read offset (chars.: 0)")) -> ("character string"=→"String Control 6":string)  [unwired: 4 in, 3 out]
          }
        }
        n2788 = case shown="True" "OPEN 4" {
          frame False {
          }
          frame True {
            (unwired) 0  # existing file
            w3603 = "Choose a datalog file to open"  # prompt
            n2789 = local write "OPEN 4"(FALSE ("OPEN 1")) -> ()
            n2790 = String To Path(string="C:\\LAB-IQ\\Data\\") -> (path=w3588:path)
            n2791 = File Dialog(6:"*.dgf" ("pattern"), 7:w3603, 11:w3588) -> (0:w3586:errorcluster, 3:w3594:path)  [unwired: 4 in, 2 out]
            n2792 = Unbundle(w3586) -> ()  [unwired: 3 out]
            n2793 = Strip Path(path=w3594) -> (name=w3592:string)  [unwired: 1 out]
            n2794 = Path To String(path=w3594) -> (string=w3589:string)
            "string1 4" <- w3589
            n2795 = Match Pattern(string=w3592, regular expression=".dgf") -> (before substring=→"String Control 7":string)  [unwired: 1 in, 3 out]
            n2796 = Match Pattern(string=w3589, regular expression=".dgf" ("substring (\"\")")) -> (before substring=w3599:string)  [unwired: 1 in, 3 out]
            n2797 = Concatenate Strings(w3599, ".duf" ("Substring")) -> (w3596:string)
            n2798 = String To Path(string=w3596) -> (path=w3600:path)
            n2799 = call <vilib>:"Read Characters From File.vi"("file path (dialog if empty)"=w3600, "start of read offset (chars.:0)"=60 ("start of read offset (chars.: 0)")) -> ("character string"=→"String Control 8":string)  [unwired: 4 in, 3 out]
          }
        }
      }
      frame "About" {
        # "Elapsed time\ncof\nstroke\nmean pos\nTemp\nHumidity"
        n2800 = disable-structure shown="Disabled" {
          frame Disabled {
            n2801 = case shown="True" "Export" {
              frame False {
              }
              frame True {
                w3625 = "                                      " ("string")
                w3627 = "\r"
                (unwired) i16 6 ("width (-)")
                w3704 = "\r"
                w3636 = "\r"
                n2802 = local write "Export"(FALSE ("Export")) -> ()
                n2803 = local read "String 29"() -> (w3673:string)
                n2804 = local read "String 34"() -> (w3661:string)
                n2805 = local read "String 35"() -> (w3656:string)
                n2806 = local read "String 37"() -> (w3652:string)
                n2807 = local read "String 36"() -> (w3649:string)
                n2808 = local read "String 38"() -> (w3646:string)
                n2809 = local read "String 39"() -> (w3643:string)
                n2810 = Match Pattern(string=w3673, regular expression=".dwm") -> (before substring=w3669:string)  [unwired: 1 in, 3 out]
                "before substring" <- w3669
                n2811 = local read "S 38"() -> (w3664:string)
                n2812 = local read "S 39"() -> (w3657:string)
                n2813 = local read "Temperature before test 2"() -> (w3693:dbl)
                n2814 = local read "Temperature after test 2"() -> (w3698:dbl)
                n2815 = local read "Humidity before test 2"() -> (w3679:dbl)
                n2816 = local read "Humidity after test 2"() -> (w3694:dbl)
                n2817 = local read "MWSD 2"() -> (w3690:dbl)
                n2818 = local read "WS1.4 2"() -> (w3706:dbl)
                n2819 = local read "HCF 2"() -> (w3702:dbl)
                n2820 = local read "AVP 2"() -> (w3691:dbl)
                n2821 = Concatenate Strings("1," ("string"), w3664) -> (w3663:string)
                n2822 = Concatenate Strings("2," ("string"), w3661) -> (w3660:string)
                n2823 = Concatenate Strings("3," ("string"), w3657) -> (w3659:string)
                n2824 = Concatenate Strings("4," ("string"), w3656) -> (w3655:string)
                n2825 = Concatenate Strings("5," ("string"), w3652) -> (w3653:string)
                n2826 = Concatenate Strings("6," ("string"), w3649) -> (w3650:string)
                n2827 = Concatenate Strings("7," ("string"), w3646) -> (w3647:string)
                n2828 = Concatenate Strings("8," ("string"), w3643) -> (w3644:string)
                n2829 = local read "Sample ID"() -> (w3711:string)
                n2830 = case shown="\"xlx\"" "Select File Type" {
                  tunnel: w3669 -> [w3714 w3716 w3718]
                  tunnel: [w3712 w3717 w3719] -> w3668
                  frame "xlx" {
                    n2831 = Concatenate Strings(w3714, ".xls" ("string")) -> (w3712:string)
                  }
                  frame "csv" {
                    n2832 = Concatenate Strings(w3716, ".csv" ("string")) -> (w3717:string)
                  }
                  frame "txt" {
                    n2833 = Concatenate Strings(w3718, ".txt" ("string")) -> (w3719:string)
                  }
                }
                n2834 = local read "Test Date"() -> (w3710:string)
                n2835 = local read "String 45"() -> (w3624:string)
                n2836 = local read "String 31"() -> (w3709:string)
                n2837 = local read "String 32"() -> (w3708:string)
                n2838 = local read "TITTLE"() -> (w3632:string)
                n2839 = Number To Fractional String(number=w3679, width (-)=i16 6, precision (6)=i16 2) -> (F-format string=w3678:string)  [unwired: 1 in]
                n2840 = Number To Fractional String(number=w3693, width (-)=i16 6, precision (6)=i16 2) -> (F-format string=w3699:string)  [unwired: 1 in]
                n2841 = Number To Fractional String(number=w3694, width (-)=i16 6, precision (6)=i16 2) -> (F-format string=w3692:string)  [unwired: 1 in]
                n2842 = Number To Fractional String(number=w3698, width (-)=i16 6, precision (6)=i16 2) -> (F-format string=w3697:string)  [unwired: 1 in]
                n2843 = Number To Fractional String(number=w3690, width (-)=i16 6, precision (6)=i16 2) -> (F-format string=w3688:string)  [unwired: 1 in]
                n2844 = Number To Fractional String(number=w3691, width (-)=i16 6, precision (6)=i16 2) -> (F-format string=w3689:string)  [unwired: 1 in]
                n2845 = Number To Fractional String(number=w3702, width (-)=i16 6, precision (6)=i16 2) -> (F-format string=w3703:string)  [unwired: 1 in]
                n2846 = Number To Fractional String(number=w3706, precision (6)=i16 2) -> (F-format string=w3707:string)  [unwired: 2 in]
                n2847 = local read "s.NO"() -> (w3626:string)
                n2848 = Concatenate Strings("=" ("string"), w3632) -> (w3631:string)
                n2849 = Concatenate Strings("S.No," ("string"), "                                       Parameters" ("string")) -> (w3637:string)
                n2850 = Concatenate Strings(w3704, w3663, w3678, w3704, w3660, w3699, w3704, w3659, w3692, w3704, w3655, w3697, w3704, w3653, w3688, w3704, w3650, w3689, w3704, w3647, w3703, w3704, w3644, w3707) -> (w3666:string)
                n2851 = Concatenate Strings(w3636, "," ("string"), w3624, w3626, w3625, w3708, w3711, w3625, w3709, w3710, w3636) -> (w3634:string)
                n2852 = local read "Tested by"() -> (w3640:string)
                n2853 = local read "String 33"() -> (w3641:string)
                n2854 = Concatenate Strings("," ("string"), "                                                                             " ("string")) -> (w3629:string)
                n2855 = Concatenate Strings(w3631, w3627, w3634, w3627, w3637, w3666, w3627, w3629, w3641, w3640) -> (→"export":string)
                n2856 = String To Path(string=w3668) -> (path=w3675:path)
                n2857 = local read "export"() -> (w3670:string)
                n2858 = call <vilib>:"Write Characters To File.vi"("append to file? (new file:F)"=FALSE, "character string"=w3670, "file path (dialog if empty)"=w3675) -> ()  [unwired: 2 in, 1 out]
              }
            }
          }
          frame Enabled {
          }
        }
        n2859 = case shown="True" "OK Button 17" {
          frame False {
          }
          frame True {
            (unwired) 0  # existing file
            w3928 = "Choose a datalog file to open"  # prompt
            n2860 = local write "OK Button 17"(FALSE ("OK Button 17")) -> ()
            n2861 = local read "String"() -> (w3923:string)
            n2862 = String To Path(string=w3923) -> (path=w3924:path)
            n2863 = File Dialog(6:"*.duf" ("pattern"), 7:w3928, 11:w3924) -> (0:w3915:errorcluster, 3:w3934:path)  [unwired: 4 in, 2 out]
            n2864 = Unbundle(w3915) -> ()  [unwired: 3 out]
            n2865 = Open/Create/Replace File "Open File"(file path (use dialog)=w3934) -> (refnum out=w3926:refnum<file>)  [unwired: 5 in, 2 out]
            n2866 = Strip Path(path=w3934) -> (name=w3932:string)  [unwired: 1 out]
            n2867 = Path To String(path=w3934) -> (string=w3917:string)
            n2868 = while {
              tunnel: w3926 -> [w3938]
              i -> [w3935]
              stop <- w3936 continue-if-true
              (unwired) TRUE ("line mode (F)")
              n2869 = Read from Text File "Read File"(file (use dialog)=w3938) -> (text=w3937:string)  [unwired: 3 in, 3 out]
              n2870 = local write "Numeric 16"(w3935) -> ()
              n2871 = String Length(string=w3937) -> (length=w3940:i32)
              n2872 = Greater?(x=w3940, y=1) -> (0:w3936:bool)
            }
            n2873 = local write "String 29"(w3917) -> ()
            n2874 = Search and Replace String(input string=w3917, search string=".duf", replace string=".dgf" ("replace string (\"\")")) -> (result string=→"String Indicator 4":string)  [unwired: 5 in, 3 out]
            n2875 = Match Pattern(string=w3932, regular expression=".dwm") -> (before substring=w3916:string)  [unwired: 1 in, 3 out]
            "String Indicator" <- w3916
            n2876 = Match Pattern(string=w3917, regular expression=".dwm" ("substring (\"\")")) -> (before substring=w3918:string)  [unwired: 1 in, 3 out]
            "String Indicator 3" <- w3918
            n2877 = local write "TITTLE 2"(w3916) -> ()
            n2878 = String To Path(string=w3918) -> (path=w3925:path)
            "path" <- w3925
            n2879 = call <vilib>:"Read Characters From File.vi"("file path (dialog if empty)"=w3925, "start of read offset (chars.:0)"=60 ("start of read offset (chars.: 0)")) -> ("character string"=→"String Indicator 2":string)  [unwired: 4 in, 3 out]
          }
        }
        n2880 = call <vilib>:"Query Available Printers.vi"() -> ("system configured printers"=w3617:string[])  [unwired: 9 in, 2 out]
        "System Configured Printers 2" <- w3617
        n2881 = local read "OK Button 16"() -> (w3614:bool)
        n2882 = case shown="True" "OK Button 16" {
          frame False {
          }
          frame True {
            n2883 = stacked-sequence {
              frame #0 {
                n2884 = local read "Numeric 16"() -> (w3942:i32)
                n2885 = local write "Numeric 10"(w3942) -> ()
              }
              frame #1 {
                n2886 = local read "String 29"() -> (w3945:string)
                n2887 = String To Path(string=w3945) -> (path=w3944:path)
                n2888 = Open/Create/Replace File "Open File"(file path (use dialog)=w3944) -> (refnum out=w3946:refnum<file>)  [unwired: 5 in, 2 out]
                n2889 = for {
                  N: 16 -> [_]
                  tunnel: w3946 -> [w3953]
                  i -> [w3949]
                  (unwired) TRUE ("line mode (F)")
                  n2890 = Read from Text File "Read File"(file (use dialog)=w3953) -> (text=w3947:string)  [unwired: 3 in, 3 out]
                  n2891 = Match Pattern(string=w3947, regular expression="(") -> (after substring=w3952:string)  [unwired: 1 in, 3 out]
                  n2892 = Match Pattern(string=w3952, regular expression=")") -> (before substring=w3948:string)  [unwired: 1 in, 3 out]
                  n2893 = case shown="1" w3949 {
                    tunnel: w3948 -> [w3954 w3955 _ _ w3956 w3957 w3958 w3960 w3962 w3964 w3966 w3968 w3970 w3972 _]
                    tunnel: w3947 -> [_ _ _ _ _ _ _ _ _ _ _ _ _ _ _]
                    frame 0 {
                      "TITTLE" <- w3954
                    }
                    frame 1 {
                      "Sample ID" <- w3955
                    }
                    frame 2 {
                    }
                    frame 3 {
                    }
                    frame 4 {
                      "Test Date" <- w3956
                    }
                    frame 5 {
                      "Tested by" <- w3957
                    }
                    frame 6 {
                      n2894 = Fract/Exp String To Number(string=w3958) -> (number=→"Humidity before test 2":dbl)  [unwired: 3 in, 1 out]
                    }
                    frame 7 {
                      n2895 = Fract/Exp String To Number(string=w3960) -> (number=→"Temperature before test 2":dbl)  [unwired: 3 in, 1 out]
                    }
                    frame 8 {
                      n2896 = Fract/Exp String To Number(string=w3962) -> (number=→"Humidity after test 2":dbl)  [unwired: 3 in, 1 out]
                    }
                    frame 9 {
                      n2897 = Fract/Exp String To Number(string=w3964) -> (number=→"Temperature after test 2":dbl)  [unwired: 3 in, 1 out]
                    }
                    frame 10 {
